vi "Log Custom Info.vi"(8 "error in (no error)":errorcluster, 9 "Write to Terminal":bool=TRUE, 10 "Custom Message":string, 11 "CIFCorePlugin in":refnum<class "CIFCorePlugin.lvclass">) -> (0 "error out":errorcluster, 3 "CIFCorePlugin out":refnum<class "CIFCorePlugin.lvclass">)   [LabVIEW 2021, in "CIFCorePlugin.lvclass"]
doc: "Log custom message into the information log and optionally display to the terminal."
uses:
  CIFCorePlugin.lvclass
  CIFCorePlugin.lvclass/CIFCorePlugin.ctl
  Accessors/Read Plugin Name.vi
  CIFUtilities/CIFLogs/CIFLogs.lvlib
  CIFUtilities/CIFLogs/Typedef/Message Type.ctl
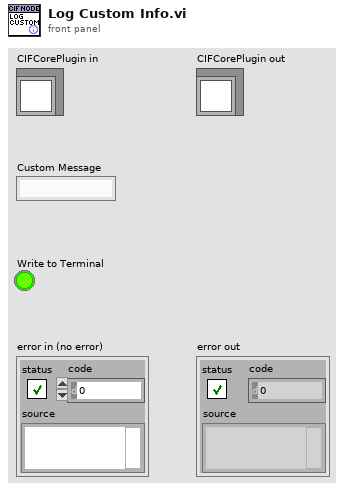
[diagram p1: front panel]
types:
  T1 = typedef "CIFLogs.lvlib/Message Type.ctl" = enum16{"Error", "Information", "Print Terminal", "Configuration"}
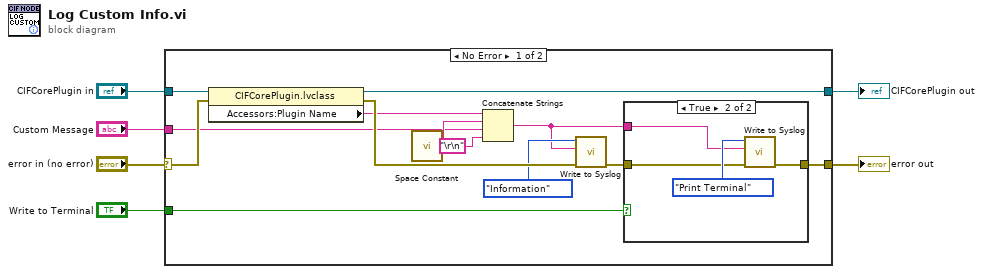
[diagram p0: block diagram]
diagram:
  n1 = case shown="No Error" "error in (no error)" {
    selector: "error in (no error)" -> [w16 w26]
    tunnel: [w14 w26] -> w5
    tunnel: [w18 w25] -> w3
    tunnel: "CIFCorePlugin in" -> [w19 w25]
    tunnel: "Custom Message" -> [w8 _]
    tunnel: "Write to Terminal" -> [w7 _]
    frame No Error {
      n2 = property class="CIFCorePlugin.lvclass"(reference=w19, error in=w16) -> (reference out=w18:refnum<class "CIFCorePlugin.lvclass">, error out=w17:errorcluster, "Accessors:Plugin Name"=w15:string)
      n3 = call <vilib>:"Space Constant.vi"() -> ("String"=w9:string)
      n4 = Concatenate Strings(w15, w9, w8, "\r\n") -> (w11:string)
      n5 = call "Write to Syslog.vi"("error in (no error)"=w17, "message"=w11, "CIF Message Type"=Message_Type."Information") -> ("error out"=w12:errorcluster)  [unwired: 8 in]
      n6 = case shown="True" w7 {
        tunnel: [w20 w24] -> w14
        tunnel: w12 -> [w20 w22]
        tunnel: w11 -> [_ w21]
        frame False {
        }
        frame True {
          n7 = call "Write to Syslog.vi"("error in (no error)"=w22, "message"=w21, "CIF Message Type"=Message_Type."Print Terminal") -> ("error out"=w24:errorcluster)  [unwired: 8 in]
        }
      }
    }
    frame Error {
    }
  }
  "error out" <- w5
  "CIFCorePlugin out" <- w3
